vi "Clear Index.vi"(8 "error in (no error)":errorcluster, 10 "Project Path":path) -> (0 "error out":errorcluster)   [LabVIEW 2020, in "Test Finder.lvclass"]
uses:
  Test Finder.lvclass
  Private/Filter Test Cases.vi
  Private/Find all Classes in LV XML.vi
  <vilib>/Utility/LVClass/Get LV Class Default Value.vi
  LUnit Test Case.lvclass
  Test Finder.lvclass/Test Finder.ctl
  User Interface/Support/Paths.lvlib
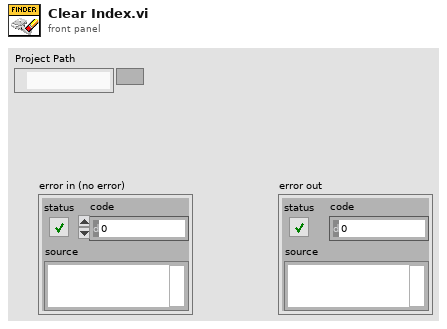
[diagram p1: front panel]
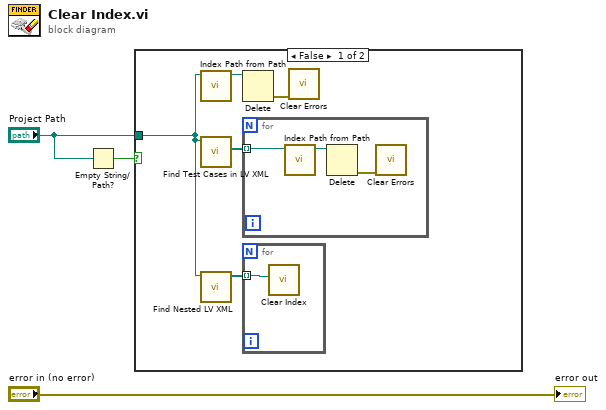
[diagram p0: block diagram]
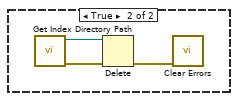
[diagram p2: hidden frame]
diagram:
  n1 = Empty String/Path?(string/path="Project Path") -> (empty?=w2:bool)
  n2 = case shown="False" w2 {
    tunnel: "Project Path" -> [w5 _]
    frame False {
      n3 = call "Index Path from Path.vi"("Project Path"=w5) -> ("appended path"=w8:path)  [unwired: 10 in]
      n4 = call "Find Test Cases in LV XML.vi"("Path"=w5) -> ("Test Class paths"=w6:path[])  [unwired: 9 in, 1 out]
      n5 = call "Find Nested LV XML.vi"("Projext Path"=w5) -> ("lvprojs"=w7:path[])  [unwired: 8 in, 2 out]
      n6 = Delete(path (use dialog)=w8) -> (error out=w4:errorcluster)  [unwired: 4 in, 2 out]
      n7 = for {
        tunnel: w6 -> [w11] mode=indexing
        n8 = call "Index Path from Path.vi"("Project Path"=w11) -> ("appended path"=w10:path)  [unwired: 10 in]
        n9 = Delete(path (use dialog)=w10) -> (error out=w9:errorcluster)  [unwired: 4 in, 2 out]
        n10 = call <vilib>:"Clear Errors.vi"("error in (no error)"=w9) -> ()  [unwired: 5 in, 2 out]
      }
      n11 = for {
        tunnel: w7 -> [w12] mode=indexing
        n12 = call "Clear Index.vi"("Project Path"=w12) -> ()  [unwired: 10 in, 1 out]
      }
      n13 = call <vilib>:"Clear Errors.vi"("error in (no error)"=w4) -> ()  [unwired: 5 in, 2 out]
    }
    frame True {
      n14 = call "Get Index Directory Path.vi"() -> ("error out"=w14:errorcluster, "Index Directory"=w15:path)  [unwired: 10 in]
      n15 = Delete(path (use dialog)=w15, error in=w14) -> (error out=w13:errorcluster)  [unwired: 3 in, 2 out]
      n16 = call <vilib>:"Clear Errors.vi"("error in (no error)"=w13) -> ()  [unwired: 5 in, 2 out]
    }
  }
  "error out" <- "error in (no error)"
